vi "User App.vi"() -> ()   [LabVIEW 2011, in "LVH-Xbox-One-Controller.lvlib"]
uses:
  LVH-Xbox-One-Controller.lvlib
  Private/Type Defs/Indicators/All Buttons Visual.ctl
  Private/Type Defs/Indicators/A.ctl
  Private/Type Defs/Indicators/B.ctl
  Private/Type Defs/Indicators/X.ctl
  Private/Type Defs/Indicators/Y.ctl
  Private/Type Defs/Indicators/Left Bumper.ctl
  Private/Type Defs/Indicators/Right Bumper.ctl
  Private/Type Defs/Indicators/View.ctl
  Private/Type Defs/Indicators/Menu.ctl
  Private/Type Defs/Indicators/Thumbstick.ctl
  Private/Type Defs/Indicators/All Axis Data.ctl
  Private/Type Defs/Indicators/DPad Enum.ctl
panel:
  out "All Axis":T1
  out "Buttons":T3
  in  "Stop Button":bool
  out "Error Out":errorcluster
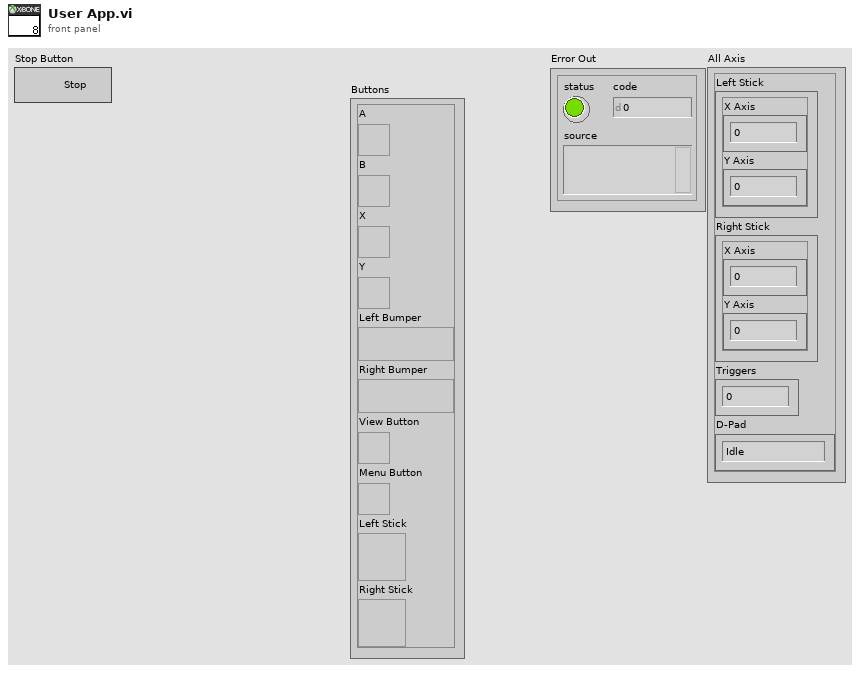
[diagram p1: front panel]
types:
  T1 = typedef "LVH-Xbox-One-Controller.lvlib/All Axis Data.ctl" = cluster{"Left Stick":cluster{"X Axis":i32, "Y Axis":i32}, "Right Stick":cluster{"X Axis":i32, "Y Axis":i32}, "Triggers":i32, "D-Pad":T2}
  T2 = typedef "LVH-Xbox-One-Controller.lvlib/DPad Enum.ctl" = enum16{"Idle", "Up", "Up / Right", "Right", "Down / Right", "Down", "Down / Left", "Left", "Up / Left"}
  T3 = typedef "LVH-Xbox-One-Controller.lvlib/All Buttons Visual.ctl" = cluster{"A":T4, "B":T5, "X":T6, "Y":T7, "Left Bumper":T8, "Right Bumper":T9, "View Button":T10, "Menu Button":T11, "Left Stick":T12, "Right Stick":T12}
  T4 = typedef "LVH-Xbox-One-Controller.lvlib/A.ctl" = bool
  T5 = typedef "LVH-Xbox-One-Controller.lvlib/B.ctl" = bool
  T6 = typedef "LVH-Xbox-One-Controller.lvlib/X.ctl" = bool
  T7 = typedef "LVH-Xbox-One-Controller.lvlib/Y.ctl" = bool
  T8 = typedef "LVH-Xbox-One-Controller.lvlib/Left Bumper.ctl" = bool
  T9 = typedef "LVH-Xbox-One-Controller.lvlib/Right Bumper.ctl" = bool
  T10 = typedef "LVH-Xbox-One-Controller.lvlib/View.ctl" = bool
  T11 = typedef "LVH-Xbox-One-Controller.lvlib/Menu.ctl" = bool
  T12 = typedef "LVH-Xbox-One-Controller.lvlib/Thumbstick.ctl" = bool
  T13 = typedef "LVH-Xbox-One-Controller.lvlib/Xbox One Controller Ref.ctl" = cluster{"Controller Ref":refnum<k1>, "Event Refnum":refnum<event-registration>, "Worker Ref":refnum<vi>}
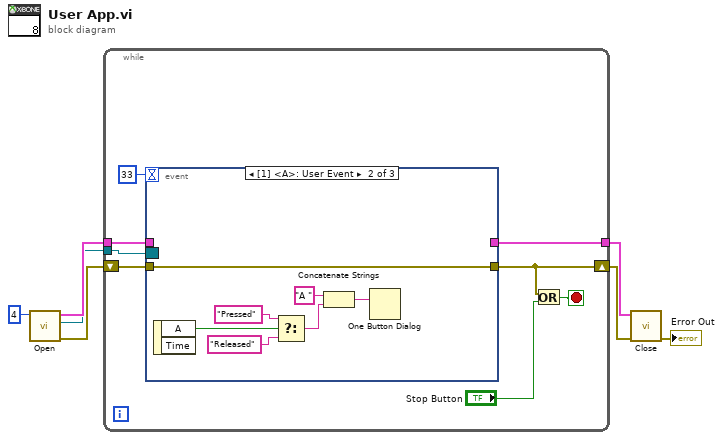
[diagram p0: block diagram]
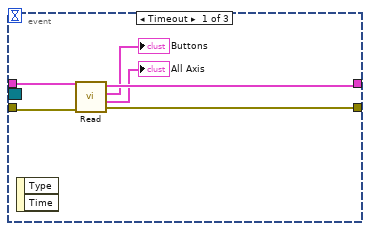
[diagram p2: hidden frame]
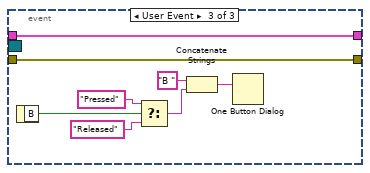
[diagram p3: hidden frame]
diagram:
  n1 = call "Open.vi"("Device Index"=4) -> ("Error Out"=w4:errorcluster, "Event Refnum"=w5:refnum<event-registration>, "Xbox One Controller Ref"=w6:T13)  [unwired: 8 in]
  n2 = while {
    tunnel: w5 -> [w8]
    shift-right: [w11] -> w3
    shift-left: w4 -> [w14]
    tunnel: w6 -> [w15]
    tunnel: [w10] -> w2
    stop <- w13 stop-if-true
    n3 = event shown="[1] <A>: User Event" {
      selector: w8 -> [_ _ _]
      dyn-events: _ -> [_ _ _]
      timeout: 33 -> [_ _ _]
      tunnel: w15 -> [w21 _ w29]
      tunnel: w14 -> [w20 w22 w30]
      tunnel: [w18 w22 w30] -> w11
      tunnel: [w19 _ w29] -> w10
      event Timeout {
        n4 = event-data() -> ()  [unwired: 1 in, 2 out]
        n5 = call "Read.vi"("Error In"=w20, "Xbox One Controller Ref"=w21) -> ("Error Out"=w18:errorcluster, "All Axis"=→"All Axis":T1, "Buttons"=→"Buttons":T3, "Xbox One Controller Ref"=w19:T13)  [unwired: 6 in]
      }
      event User Event {
        n6 = event-data() -> ("A"=w28:bool)  [unwired: 1 in, 1 out]
        n7 = Select(t="Pressed" ("string"), s=w28, f="Released" ("string")) -> (s? t:f=w23:string)
        n8 = Concatenate Strings("A " ("string"), w23) -> (w27:string)
        n9 = One Button Dialog(message=w27) -> ()  [unwired: 1 in, 1 out]
      }
      event User Event {
        n10 = event-data() -> ("B"=w31:bool)  [unwired: 1 in]
        n11 = Select(t="Pressed" ("string"), s=w31, f="Released" ("string")) -> (s? t:f=w32:string)
        n12 = Concatenate Strings("B " ("string"), w32) -> (w36:string)
        n13 = One Button Dialog(message=w36) -> ()  [unwired: 1 in, 1 out]
      }
    }
    n14 = Or(x=w11, y="Stop Button") -> (x .or. y?=w13:bool)
  }
  n15 = call "Close.vi"("Error In"=w3, "Xbox One Controller Ref"=w2) -> ("Error Out"=→"Error Out":errorcluster)  [unwired: 9 in]
